vi "PLL_Sub.vi"(9 "Allowance":dbl=0.1, 10 "Sig":waveform(dbl)={"t0"=timestamp(3571029165.757511 s since 1904-01-01), "dt"=1.9999999999999998e-05, "Y"=array[5000 elements]}, 11 "Ref":waveform(dbl)={"t0"=timestamp(3571029165.757511 s since 1904-01-01), "dt"=1.9999999999999998e-05, "Y"=array[5000 elements]}) -> (2 "Sig Out Feed through":waveform(dbl)={"t0"=timestamp(3571029165.757511 s since 1904-01-01), "dt"=1.9999999999999998e-05, "Y"=array[5000 elements]} caption="Sig", 3 "Ref_PLL_Out":waveform(dbl)={"t0"=timestamp(4.699999999999999 s since 1904-01-01), "dt"=1.9999999999999998e-05, "Y"=array[5000 elements]})   [LabVIEW 2016]
doc: "This VI adjusts both frequency and phase of one of the signals to be synchronized with the second one."
uses:
  <vilib>/measure/matone.llb/Extract Single Tone Information 1 Chan.vi
  <vilib>/Analysis/NI_AALPro.lvlib
  <vilib>/measure/NI_MAPro.lvlib
  <vilib>/measure/NI_MABase.lvlib
panel:
  out "detected phase (deg)":dbl=87.4534599760675
  out "数値":i32=47
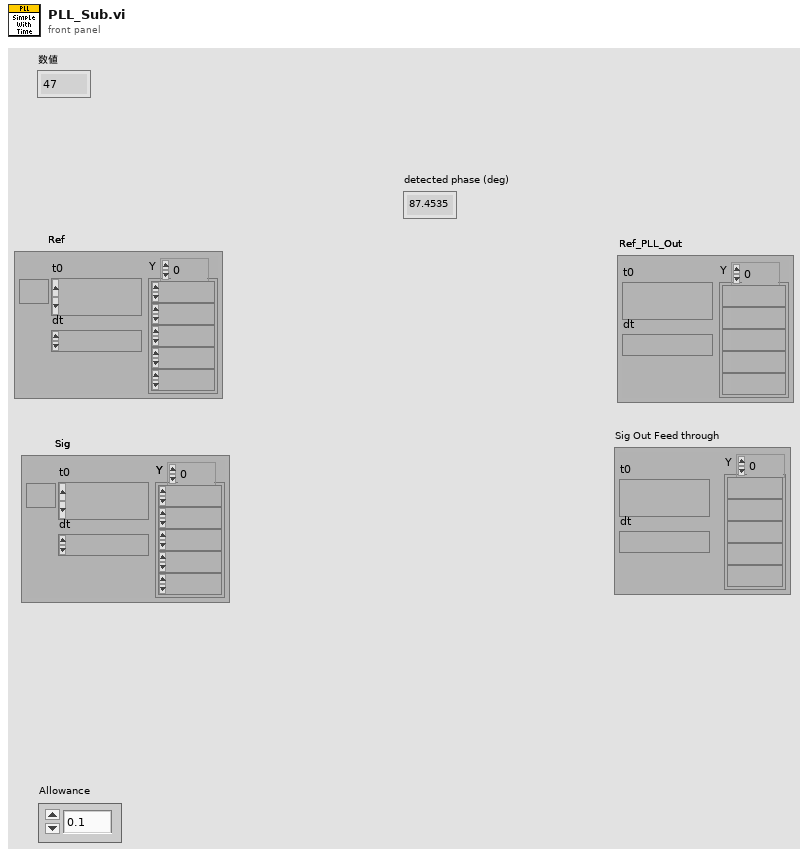
[diagram p1: front panel]
types:
  T1 = enum16{"Sine Wave", "Triangle Wave", "Square Wave", "Sawtooth Wave"}
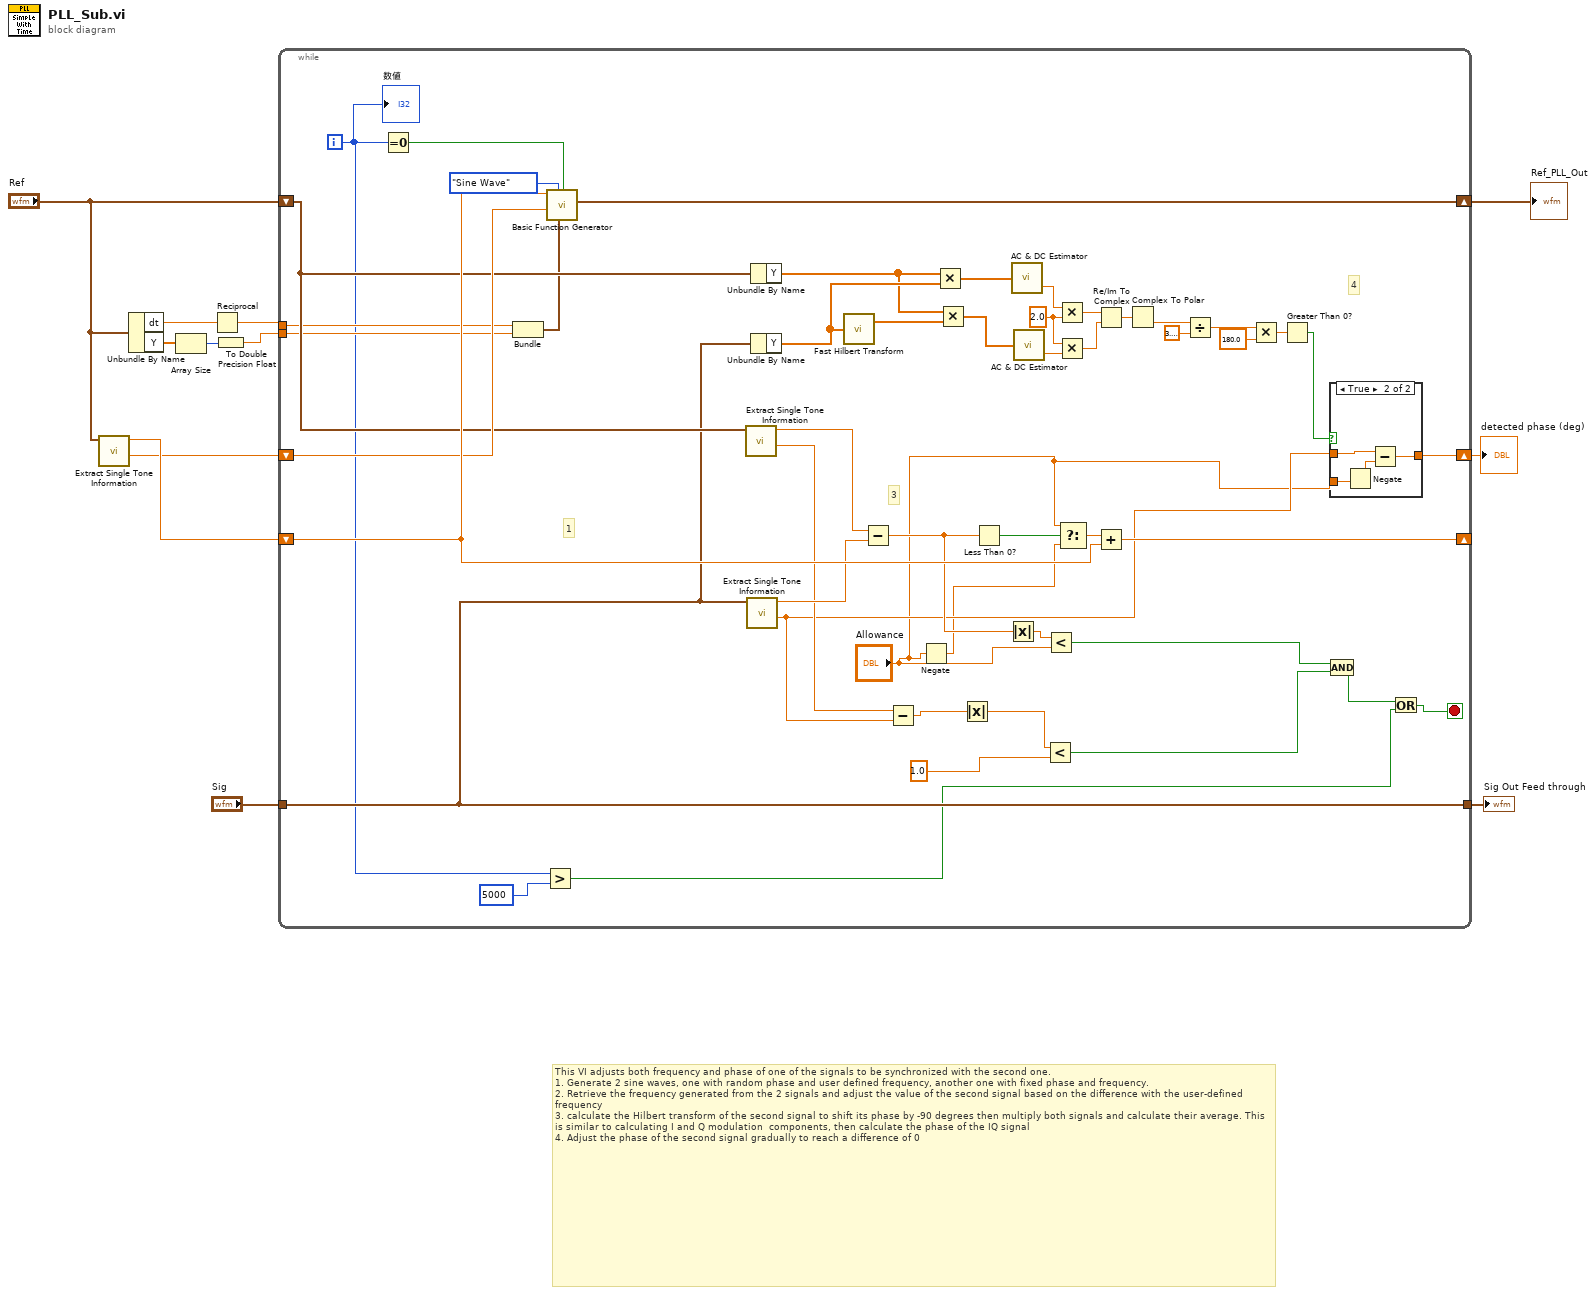
[diagram p0: block diagram]
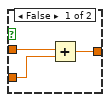
[diagram p2: hidden frame]
diagram:
  # "This VI adjusts both frequency and phase of one of the signals to be synchronized with the second one.\n1. Generate 2 sine waves, one with random phase and user defined frequency, another one with fixed phase and frequency.\n2. Retrieve the frequency generated from the 2 signals and adjust the value of the second signal based on the difference with the user-defined frequency\n3. calculate the Hilbert transform of the second signal to shift its phase by -90 degrees then multiply both signals and calculate their average. This is similar to calculating I and Q modulation  components, then calculate the phase of the IQ signal\n4. Adjust the phase of the second signal gradually to reach a difference of 0"
  n1 = call-poly <vilib>:"Extract Single Tone Information.vi"("time signal in"="Ref") -> ("detected phase (deg)"=w2:dbl, "detected frequency"=w3:dbl)  [unwired: 5 in, 4 out]
  n2 = Unbundle By Name("Ref") -> ("dt"=w8:dbl, "Y"=w7:dbl[])
  n3 = Array Size(array=w7) -> (size(s)=w9:i32)
  n4 = Reciprocal(x=w8) -> (1/x=w6:dbl)
  n5 = To Double Precision Float(number=w9) -> (double precision float=w5:dbl)
  n6 = while {
    shift-right: [w45] -> w1
    shift-left: w2 -> [w37]
    shift-right: [w58] -> _
    shift-left: w3 -> [w59]
    tunnel: "Sig" -> [w20]
    shift-right: [w21] -> w11
    shift-left: "Ref" -> [w33]
    tunnel: [w20] -> w10
    tunnel: w6 -> [w31]
    tunnel: w5 -> [w30]
    i -> [w18]
    stop <- w15 stop-if-true
    w40 = 2.0 ("x")
    # "4"
    # "3"
    # "1"
    n7 = Equal To 0?(x=w18) -> (x = 0?=w22:bool)
    n8 = Bundle(w31, w30) -> (w32:cluster{dbl, dbl})  [unwired: 1 in]
    n9 = Greater?(x=w18, y=5000) -> (0:w16:bool)
    n10 = call <vilib>:"Basic Function Generator.vi"("reset signal"=w22, "sampling info"=w32, "signal type"=T1."Sine Wave", "phase"=w37, "frequency"=w59) -> ("signal out"=w21:waveform(dbl))  [unwired: 4 in, 2 out]
    n11 = call-poly <vilib>:"Extract Single Tone Information.vi"("time signal in"=w33) -> ("detected phase (deg)"=w29:dbl, "detected frequency"=w44:dbl)  [unwired: 5 in, 4 out]
    n12 = call-poly <vilib>:"Extract Single Tone Information.vi"("time signal in"=w20) -> ("detected phase (deg)"=w28:dbl, "detected frequency"=w43:dbl)  [unwired: 5 in, 4 out]
    n13 = Unbundle By Name(w33) -> ("Y"=w55:dbl[])
    n14 = Unbundle By Name(w20) -> ("Y"=w57:dbl[])
    n15 = call <vilib>:"Fast Hilbert Transform.vi"("X"=w57) -> ("Hilbert{X}"=w56:dbl[])  [unwired: 1 out]
    n16 = Subtract(x=w44, y=w43) -> (x-y=w36:dbl)
    n17 = Subtract(x=w29, y=w28) -> (x-y=w27:dbl)
    n18 = Negate(x="Allowance") -> (-x=w14:dbl)
    n19 = Multiply(x=w55, y=w57) -> (x*y=w39:dbl[])
    n20 = Multiply(x=w55, y=w56) -> (x*y=w38:dbl[])
    n21 = Absolute Value(x=w27) -> (abs(x)=w26:dbl)
    n22 = Less Than 0?(x=w36) -> (x < 0?=w61:bool)
    n23 = Absolute Value(x=w36) -> (abs(x)=w35:dbl)
    n24 = call <vilib>:"AC & DC Estimator.vi"("Signal (V)"=w39) -> ("DC estimate (V)"=w41:dbl)  [unwired: 1 out]
    n25 = call <vilib>:"AC & DC Estimator.vi"("Signal (V)"=w38) -> ("DC estimate (V)"=w54:dbl)  [unwired: 1 out]
    n26 = Less?(x=w26, y=1.0) -> (x < y?=w24:bool)
    n27 = Less?(x=w35, y="Allowance") -> (x < y?=w34:bool)
    n28 = Multiply(x=w41, y=w40) -> (x*y=w48:dbl)
    n29 = Multiply(x=w40, y=w54) -> (x*y=w47:dbl)
    n30 = Select(t="Allowance", s=w61, f=w14) -> (s? t:f=w60:dbl)
    n31 = Re/Im To Complex(1:w47, 2:w48) -> (0:w49:cdb)
    n32 = Add(x=w60, y=w59) -> (x+y=w58:dbl)
    n33 = Complex To Polar(r * e^(i*theta)=w49) -> (theta=w50:dbl)  [unwired: 1 out]
    n34 = Divide(x=w50, y=3.141592653589793) -> (x/y=w52:dbl)
    n35 = Multiply(x=w52, y=180.0) -> (x*y=w42:dbl)
    n36 = Greater Than 0?(x=w42) -> (x > 0?=w46:bool)
    n37 = case shown="TRUE" w46 {
      tunnel: w28 -> [w63 w68]
      tunnel: [w64 w67] -> w45
      tunnel: "Allowance" -> [w62 w66]
      frame False {
        n38 = Add(x=w63, y=w62) -> (x+y=w64:dbl)
      }
      frame True {
        n39 = Negate(x=w66) -> (-x=w65:dbl)
        n40 = Subtract(x=w68, y=w65) -> (x-y=w67:dbl)
      }
    }
    n41 = Compound Arithmetic op=AND ("複合演算")(w34, w24) -> (w19:bool)
    n42 = Or(x=w19, y=w16) -> (x .or. y?=w15:bool)
    "数値" <- w18
  }
  "Ref_PLL_Out" <- w11
  "Sig Out Feed through" <- w10
  "detected phase (deg)" <- w1
